vi "Send stack info.vi"(8 "error in (no error)":errorcluster, 11 "Tomo in":refnum<class "Tomo.lvclass">) -> (0 "error out":errorcluster, 3 "Tomo out":refnum<class "Tomo.lvclass">)   [LabVIEW 2012, in "Tomo.lvclass"]
uses:
  Tomo.lvclass
  <vilib>/Distrio/Murmex/Murmex/update_cluster.ctl
  Tomo.lvclass/Tomo.ctl
  <vilib>/Distrio/Murmex/Murmex/Murmex.lvclass
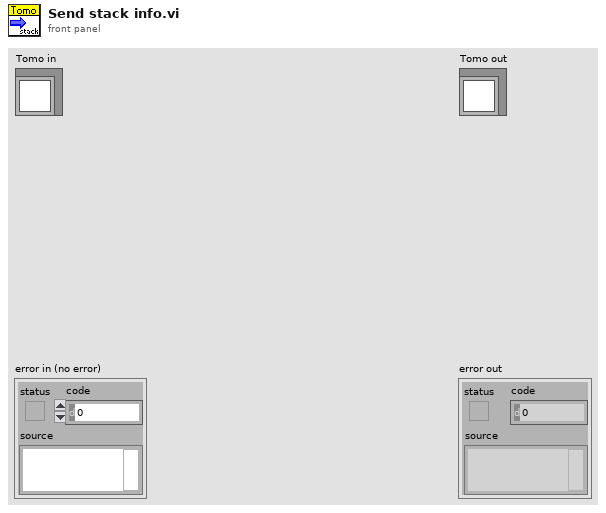
[diagram p1: front panel]
types:
  T1 = typedef "Murmex.lvlib/Murmex.lvclass/update_cluster.ctl" = cluster{"target ID":string, "key chains":string[], "values":variant[]}
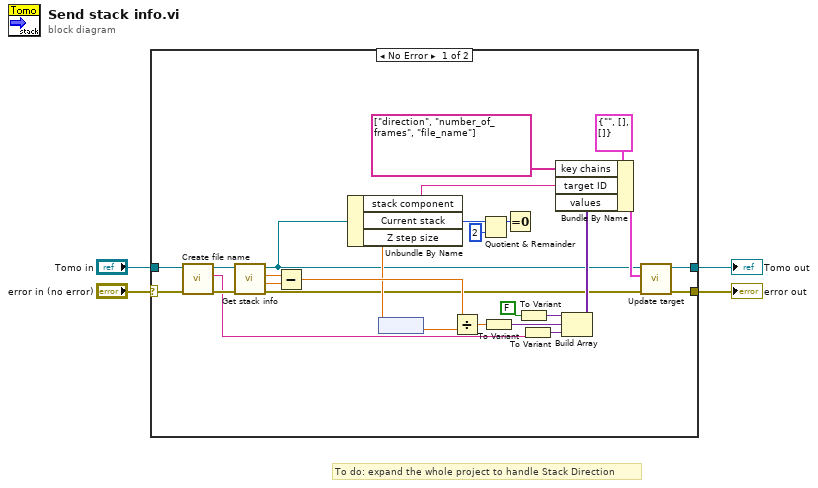
[diagram p0: block diagram]
diagram:
  # "To do: expand the whole project to handle Stack Direction"
  n1 = case shown="No Error" "error in (no error)" {
    selector: "error in (no error)" -> [w12 w33]
    tunnel: [w21 w33] -> w3
    tunnel: [w19 w32] -> w1
    tunnel: "Tomo in" -> [w10 w32]
    frame No Error {
      n2 = call-dynamic "Create file name.vi"("error in (no error)"=w12, "Tomo in"=w10) -> ("error out"=w11:errorcluster, "filename"=w7:string, "Tomo out"=w9:refnum<class "Tomo.lvclass">)  [unwired: 7 in]
      n3 = call-dynamic "Get stack info.vi"("error in (no error)"=w11, "Tomo in"=w9) -> ("error out"=w22:errorcluster, "Z start"=w30:dbl, "Z stop"=w31:dbl, "Tomo out"=w20:refnum<class "Tomo.lvclass">)  [unwired: 4 in, 2 out]
      n4 = Subtract(x=w31, y=w30) -> (x-y=w29:dbl)
      n5 = Unbundle By Name(w20) -> ("stack component"=w17:string, "Current stack"=w16:u16, "Z step size"=w28:dbl[unit])
      n6 = node(w28) -> (w5:dbl)
      n7 = Divide(x=w29, y=w5) -> (x/y=w23:dbl)
      n8 = Quotient & Remainder(x=w16, y=u16 2) -> (x-y*floor(x/y)=w13:u16)  [unwired: 1 out]
      n9 = To Variant(anything=w23) -> (Variant=w26:variant)
      n10 = Equal To 0?(x=w13) -> ()  [unwired: 1 out]
      n11 = To Variant(anything=FALSE ("x = 0?")) -> (Variant=w14:variant)
      n12 = To Variant(anything=w7) -> (Variant=w8:variant)
      n13 = Build Array(w14, w26, w8) -> (w25:variant[])
      n14 = Bundle By Name(cluster=T1 {"target ID"="", "key chains"=[], "values"=[]} ("update cluster"), "key chains"=string[] ["direction", "number_of_frames", "file_name"], "target ID"=w17, "values"=w25) -> (w27:T1)
      n15 = call <vilib>:"Update target.vi"("error in (no error)"=w22, "update cluster"=w27, "MurmexBase in"=w20) -> ("error out"=w21:errorcluster, "MurmexBase out"=w19:refnum<class "Tomo.lvclass">)  [unwired: 7 in]
    }
    frame Error {
    }
  }
  "error out" <- w3
  "Tomo out" <- w1
